vi "Ticks Per Second to RPM.vi"(10 "Ticks per Rotation":dbl, 11 "Ticks Per Second":dbl) -> (3 "RPM":dbl)   [LabVIEW 2015]
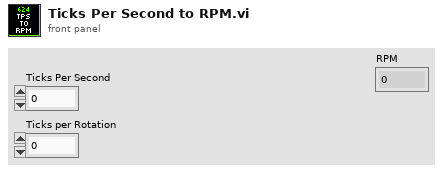
[diagram p1: front panel]
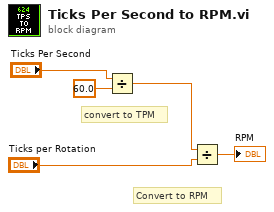
[diagram p0: block diagram]
diagram:
  # "Convert to RPM"
  # "convert to TPM"
  n1 = Divide(x="Ticks Per Second", y=60.0) -> (x/y=w3:dbl)
  n2 = Divide(x=w3, y="Ticks per Rotation") -> (x/y=→"RPM":dbl)
